vi "GlobalGetAvantesSpectrometerOnOff.vi"() -> ()   [LabVIEW 2013]
panel:
  out "GetAvantes":bool
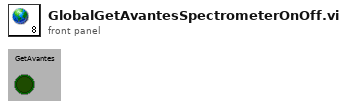
[diagram p1: front panel]
diagram:
